vi "Replace Enqueue if Using PPL.vi"(8 "error in (no error)":errorcluster, 10 "Target":refnum<vi>, 11 "Send VI ref in":refnum<vi>) -> (0 "error out":errorcluster, 3 "Send VI ref out":refnum<vi>)   [LabVIEW 2020, in "Message Maker.lvlib"]
uses:
  Message Maker.lvlib
  <vilib>/Utility/traverseref.llb/TRef TravTarget.ctl
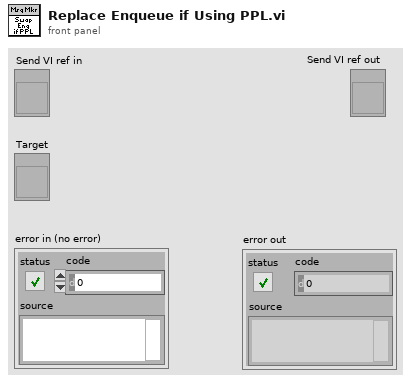
[diagram p1: front panel]
types:
  T1 = typedef "TRef TravTarget.ctl" = enum16{"FP", "BD", "Other"}
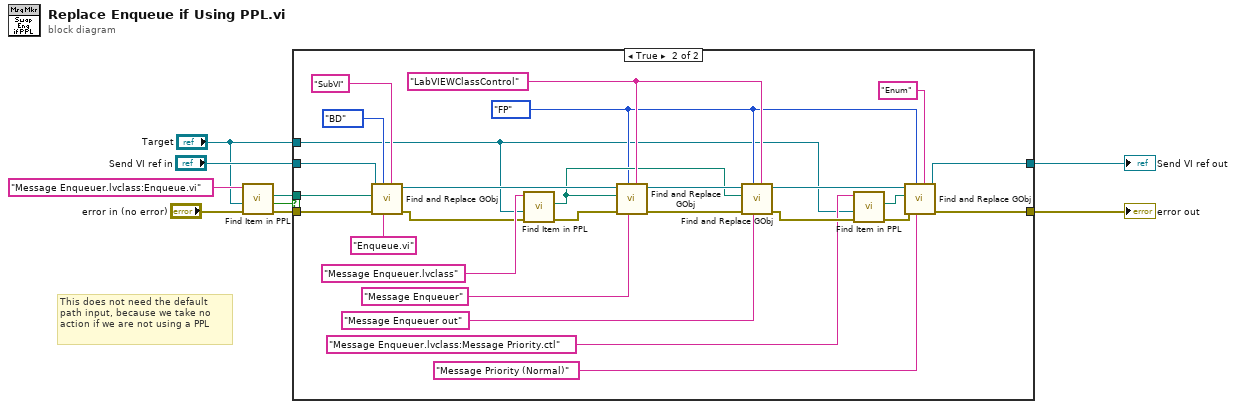
[diagram p0: block diagram]
diagram:
  # "This does not need the default path input, because we take no action if we are not using a PPL"
  n1 = call "Find Item in PPL.vi"("error in (no error)"="error in (no error)", "Target"="Target", "qualified name"="Message Enqueuer.lvclass:Enqueue.vi") -> ("error out"=w8:errorcluster, "ppl exists?"=w3:bool, "item path out"=w5:path)  [unwired: 6 in]
  n2 = case shown="True" w3 {
    tunnel: w8 -> [w10 w38]
    tunnel: "Send VI ref in" -> [w11 w37]
    tunnel: [w11 w14] -> w6
    tunnel: w5 -> [_ w34]
    tunnel: [w10 w13] -> w2
    tunnel: "Target" -> [_ w12]
    frame False {
    }
    frame True {
      w16 = TRef_TravTarget."FP" ("Traverse Target")
      w27 = "LabVIEWClassControl" ("Class Name")
      n3 = call "Find and Replace GObj.vi"("GObj Class Name"="SubVI", "GObj Label"="Enqueue.vi", "Traverse Target"=TRef_TravTarget."BD", "error in (no error)"=w38, "Class Path"=w34, "vi reference in"=w37) -> ("error out"=w22:errorcluster, "vi reference out"=w32:refnum<vi>)  [unwired: 3 in, 1 out]
      n4 = call "Find Item in PPL.vi"("error in (no error)"=w22, "Target"=w12, "qualified name"="Message Enqueuer.lvclass") -> ("error out"=w30:errorcluster, "item path out"=w26:path)  [unwired: 6 in, 1 out]
      n5 = call "Find and Replace GObj.vi"("GObj Class Name"=w27, "GObj Label"="Message Enqueuer", "Traverse Target"=w16, "error in (no error)"=w30, "Class Path"=w26, "vi reference in"=w32) -> ("error out"=w23:errorcluster, "vi reference out"=w31:refnum<vi>)  [unwired: 3 in, 1 out]
      n6 = call "Find and Replace GObj.vi"("GObj Class Name"=w27, "GObj Label"="Message Enqueuer out", "Traverse Target"=w16, "error in (no error)"=w23, "Class Path"=w26, "vi reference in"=w31) -> ("error out"=w21:errorcluster, "vi reference out"=w24:refnum<vi>)  [unwired: 3 in, 1 out]
      n7 = call "Find Item in PPL.vi"("error in (no error)"=w21, "Target"=w12, "qualified name"="Message Enqueuer.lvclass:Message Priority.ctl") -> ("error out"=w19:errorcluster, "item path out"=w18:path)  [unwired: 6 in, 1 out]
      n8 = call "Find and Replace GObj.vi"("GObj Class Name"="Enum", "GObj Label"="Message Priority (Normal)", "Traverse Target"=w16, "error in (no error)"=w19, "Class Path"=w18, "vi reference in"=w24) -> ("error out"=w13:errorcluster, "vi reference out"=w14:refnum<vi>)  [unwired: 3 in, 1 out]
    }
  }
  "Send VI ref out" <- w6
  "error out" <- w2
